vi "Read Calibration Release 1.vi"(6 "error in":errorcluster, 8 "MaxRead":i32, 9 "Channel in":u16) -> (0 "error out":errorcluster, 1 "Messages":T1(array[cluster]), 2 "Pass":bool, 3 "Channel out":u16, 4 "Calibration Release Number":string)   [LabVIEW 2023]
uses:
  4f930f32-d09a-43ef-bca1-8b214b378bd5.vi
  e8470de1-fa2d-4ee3-b50e-96bd89dc731f.vi
  d0f02419-cfb7-4a5e-bc3c-f035efdb0e96.vi
  Communication/PCAN2023/PCAN API.lvlib
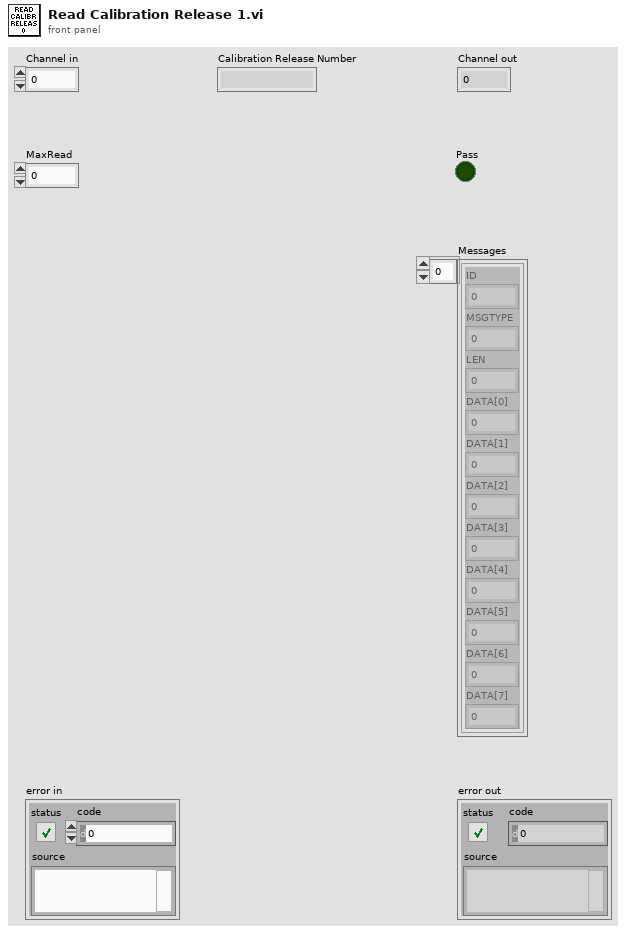
[diagram p1: front panel]
types:
  T1 = cluster{"ID":u32, "MSGTYPE":u8, "LEN":u8, "DATA[0]":u8, "DATA[1]":u8, "DATA[2]":u8, "DATA[3]":u8, "DATA[4]":u8, "DATA[5]":u8, "DATA[6]":u8, "DATA[7]":u8}[]
  T2 = cluster{"ID":u32, "MSGTYPE":u8, "LEN":u8, "DATA[0]":u8, "DATA[1]":u8, "DATA[2]":u8, "DATA[3]":u8, "DATA[4]":u8, "DATA[5]":u8, "DATA[6]":u8, "DATA[7]":u8}
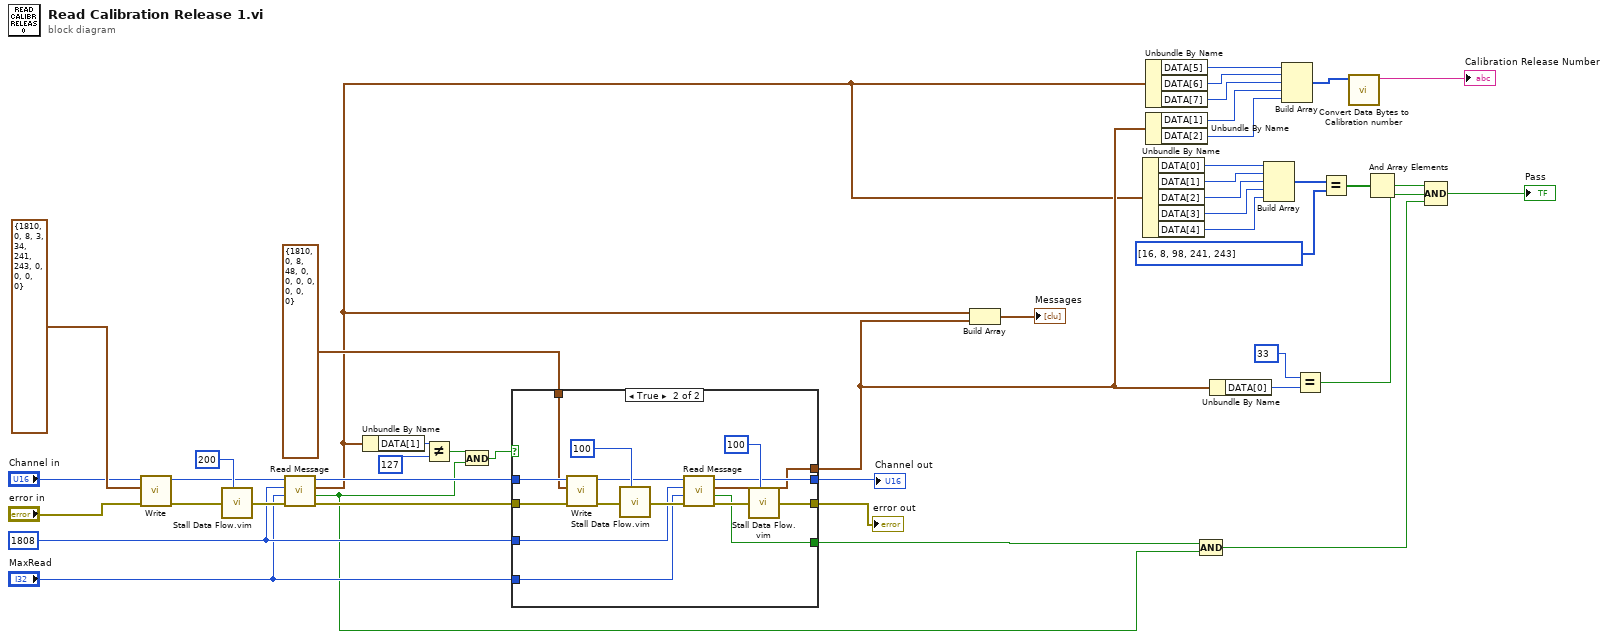
[diagram p0: block diagram]
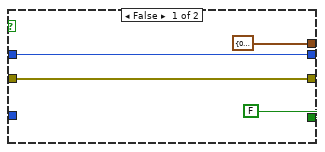
[diagram p2: hidden frame]
diagram:
  (unwired) u32 200 ("milliseconds to wait")
  w8 = u32 1808 ("ID")
  n1 = call "Write.vi"("error in"="error in", "MessageBuffer"=T2 {"ID"=1810, "MSGTYPE"=0, "LEN"=8, "DATA[0]"=3, "DATA[1]"=34, "DATA[2]"=241, "DATA[3]"=243, "DATA[4]"=0, "DATA[5]"=0, "DATA[6]"=0, "DATA[7]"=0}, "Channel"="Channel in") -> ("error out"=w40:errorcluster, "Channel out"=w13:u16)  [unwired: 5 in, 2 out]
  n2 = call "Stall Data Flow.vim"("value in"=w40, "milliseconds to wait"=u32 200) -> ("value out"=w11:errorcluster)  [unwired: 1 out]
  n3 = call "Read Message.vi"("error in"=w11, "MaxRead"="MaxRead", "ID"=w8, "Channel in"=w13) -> ("error out"=w10:errorcluster, "Passed"=w2:bool, "Last Message"=w9:T2, "Channel out"=w12:u16)  [unwired: 3 in, 1 out]
  n4 = Unbundle By Name(w9) -> ("DATA[1]"=w35:u8)
  n5 = Not Equal?(x=w35, y=u8 127) -> (x != y?=w3:bool)
  n6 = And(x=w3, y=w2) -> (x .and. y?=w1:bool)
  n7 = case shown="True" w1 {
    tunnel: w12 -> [w47 w63]
    tunnel: w10 -> [w45 w62]
    tunnel: [w45 w61] -> w39
    tunnel: [FALSE w51] -> w38
    tunnel: [w47 w55] -> w37
    tunnel: T2 {"ID"=1810, "MSGTYPE"=0, "LEN"=8, "DATA[0]"=48, "DATA[1]"=0, "DATA[2]"=0, "DATA[3]"=0, "DATA[4]"=0, "DATA[5]"=0, "DATA[6]"=0, "DATA[7]"=0} ("MessageBuffer") -> [_ w60]
    tunnel: [T2 {"ID"=0, "MSGTYPE"=0, "LEN"=0, "DATA[0]"=0, "DATA[1]"=0, "DATA[2]"=0, "DATA[3]"=0, "DATA[4]"=0, "DATA[5]"=0, "DATA[6]"=0, "DATA[7]"=0} w52] -> w15
    tunnel: w8 -> [_ w50]
    tunnel: "MaxRead" -> [_ w49]
    frame False {
    }
    frame True {
      n8 = call "Write.vi"("error in"=w62, "MessageBuffer"=w60, "Channel"=w63) -> ("error out"=w58:errorcluster, "Channel out"=w56:u16)  [unwired: 5 in, 2 out]
      n9 = call "Stall Data Flow.vim"("value in"=w58, "milliseconds to wait"=u32 100) -> ("value out"=w54:errorcluster)  [unwired: 1 out]
      n10 = call "Read Message.vi"("error in"=w54, "MaxRead"=w49, "ID"=w50, "Channel in"=w56) -> ("error out"=w53:errorcluster, "Passed"=w51:bool, "Last Message"=w52:T2, "Channel out"=w55:u16)  [unwired: 3 in, 1 out]
      n11 = call "Stall Data Flow.vim"("value in"=w53, "milliseconds to wait"=u32 100) -> ("value out"=w61:errorcluster)  [unwired: 1 out]
    }
  }
  "error out" <- w39
  "Channel out" <- w37
  n12 = Build Array(w9, w15) -> (→"Messages":T1)
  n13 = Unbundle By Name(w9) -> ("DATA[0]"=w32:u8, "DATA[1]"=w31:u8, "DATA[2]"=w30:u8, "DATA[3]"=w29:u8, "DATA[4]"=w28:u8)
  n14 = Unbundle By Name(w9) -> ("DATA[5]"=w20:u8, "DATA[6]"=w19:u8, "DATA[7]"=w18:u8)
  n15 = Unbundle By Name(w15) -> ("DATA[1]"=w17:u8, "DATA[2]"=w4:u8)
  n16 = Compound Arithmetic op=AND(w38, w2) -> (w14:bool)
  n17 = Unbundle By Name(w15) -> ("DATA[0]"=w25:u8)
  n18 = Build Array(w32, w31, w30, w29, w28) -> (w27:u8[])
  n19 = Build Array(w20, w19, w18, w17, w4) -> (w6:u8[])
  n20 = Equal?(x=u8 33, y=w25) -> (x = y?=w22:bool)
  n21 = Equal?(x=w27, y=u8[] [16, 8, 98, 241, 243]) -> (x = y?=w23:bool[])
  n22 = call "Convert Data Bytes to Calibration number.vi"("Data Bytes"=w6) -> ("Calibration Release Number"=→"Calibration Release Number":string)  [unwired: 10 in]
  n23 = And Array Elements(Boolean array=w23) -> (logical AND=w21:bool)
  n24 = Compound Arithmetic op=AND(w21, w22, w14) -> (→"Pass":bool)
